vi "Add Dynamic to Static Dispatch Mappings.vi"(8 "error in (no error)":errorcluster, 10 "rename data in":T1, 11 "project classes in":refnum<vi>[](array[refnum])) -> (0 "error out":errorcluster, 2 "rename metadata out":T1, 3 "project classes out":refnum<vi>[](array[refnum]))   [LabVIEW 2020, in "MeasurementService Editor.lvlib"]
uses:
  MeasurementService Editor.lvlib
  Rename Refactor Data.ctl
  Rename Refactor Mapping Info.ctl
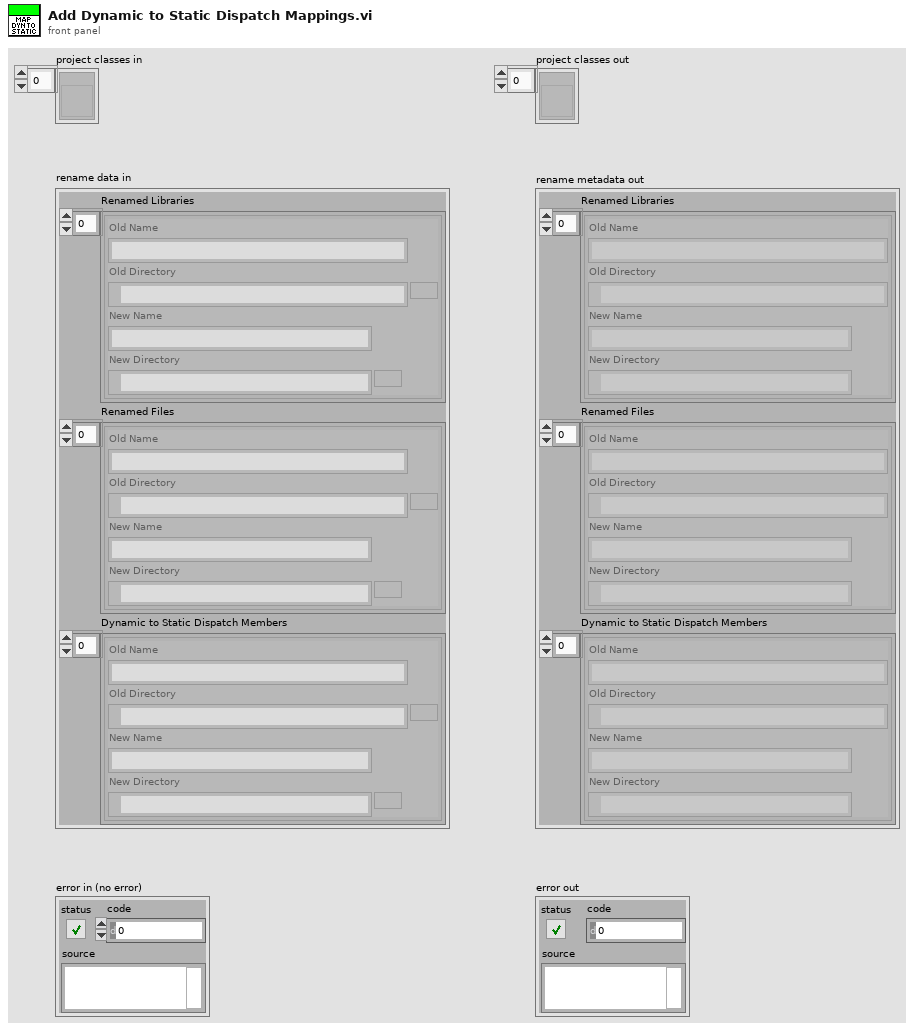
[diagram p1: front panel]
types:
  T1 = typedef "MeasurementService Editor.lvlib/Rename Refactor Data.ctl" = cluster{"Renamed Libraries":T2[], "Renamed Files":T2[], "Dynamic to Static Dispatch Members":T2[]}
  T2 = typedef "MeasurementService Editor.lvlib/Rename Refactor Mapping Info.ctl" = cluster{"Old Name":string, "Old Directory":path, "New Name":string, "New Directory":path}
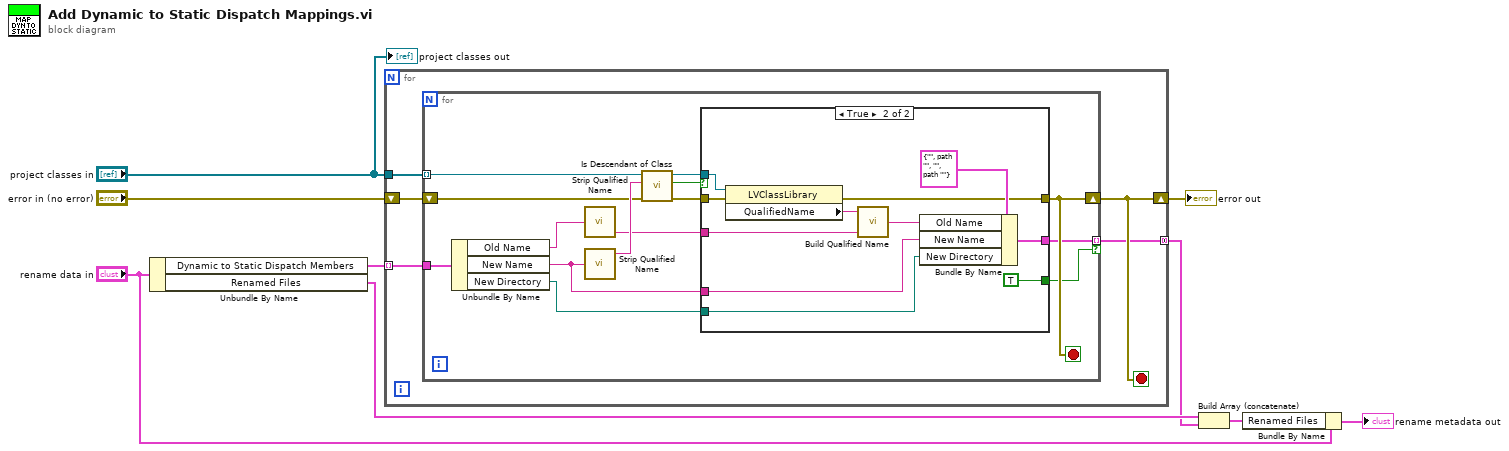
[diagram p0: block diagram]
diagram:
  n1 = Unbundle By Name("rename data in") -> ("Dynamic to Static Dispatch Members"=w8:T2[], "Renamed Files"=w6:T2[])
  n2 = for {
    tunnel: "project classes in" -> [w13]
    tunnel: w8 -> [w12] mode=indexing
    shift-right: [w11] -> w7
    shift-left: "error in (no error)" -> [w14]
    tunnel: [w10] -> w5 mode=concatenating
    stop <- w11 stop-if-true
    n3 = for {
      tunnel: w13 -> [w24] mode=indexing
      tunnel: w12 -> [w28]
      shift-right: [w17] -> w11
      shift-left: w14 -> [w25]
      tunnel: [w16] -> w10 mode=indexing if=w15
      stop <- w17 stop-if-true
      n4 = Unbundle By Name(w28) -> ("Old Name"=w27:string, "New Name"=w18:string, "New Directory"=w19:path)
      n5 = call "Strip Qualified Name.vi"("name"=w27) -> ("last name"=w21:string)  [unwired: 5 in, 1 out]
      n6 = call "Strip Qualified Name.vi"("name"=w18) -> ("stripped name"=w26:string)  [unwired: 5 in, 1 out]
      n7 = call "Is Descendant of Class.vi"("error in (no error)"=w25, "ancestor name"=w26, "class in"=w24) -> ("error out"=w22:errorcluster, "is descendant?"=w23:bool, "class out"=w20:refnum<vi>)  [unwired: 6 in]
      n8 = case shown="True" w23 {
        tunnel: w22 -> [w29 w39]
        tunnel: w21 -> [_ w36]
        tunnel: w20 -> [_ w38]
        tunnel: w19 -> [_ w33]
        tunnel: w18 -> [_ w34]
        tunnel: [_ w32] -> w16
        tunnel: [w29 w31] -> w17
        tunnel: [_ TRUE] -> w15
        frame False {
        }
        frame True {
          n9 = property class="LVClassLibrary"(reference=w38, error in=w39) -> (error out=w31:errorcluster, "QualifiedName"=w37:string)  [unwired: 1 out]
          n10 = call "Build Qualified Name.vi"("name"=w36, "base name"=w37) -> ("appended name"=w35:string)  [unwired: 3 in]
          n11 = Bundle By Name(cluster=T2 {"Old Name"="", "Old Directory"=path "", "New Name"="", "New Directory"=path ""} ("Rename Mapping Info"), "Old Name"=w35, "New Name"=w34, "New Directory"=w33) -> (w32:T2)
        }
      }
    }
  }
  "error out" <- w7
  n12 = Build Array (concatenate)(w6, w5) -> (w3:T2[])
  n13 = Bundle By Name(cluster="rename data in", "Renamed Files"=w3) -> (→"rename metadata out":T1)
  "project classes out" <- "project classes in"
